vi "Compile with Data.vi"(6 "Loader":refnum<class "Loader.lvclass">, 7 "Data":refnum<class "Datum.lvclass">=refnum, 8 "Error In":errorcluster, 11 "Input":string) -> (0 "Error Out":errorcluster, 3 "Output":string)   [LabVIEW 2018, in "Toolkit.lvlib"]
doc: "Compile a Mustache template as a string using the types of data passed into the compiler to control the how and what is provided in the output. The type fo data for each tag and key can determine the rendering behavior of the node in the syntax tree, so LabVIEW classes are provided to represent the different types of data."
uses:
  Toolkit.lvlib
  Data/Datum/Datum.lvclass
  Data/Map/Map.lvclass
  Low-Level/Loaders/Loader/Loader.lvclass
  Low-Level/Support/Lex String.vi
  Low-Level/Support/Render to String.vi
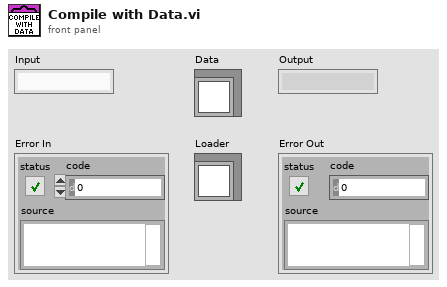
[diagram p1: front panel]
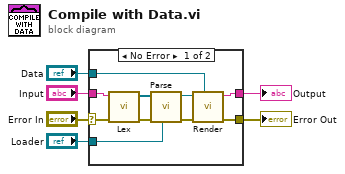
[diagram p0: block diagram]
diagram:
  n1 = case shown="No Error" "Error In" {
    selector: "Error In" -> [w10 w17]
    tunnel: [w13 w17] -> w6
    tunnel: "Input" -> [w9 w18]
    tunnel: [w12 w18] -> w4
    tunnel: "Data" -> [w11 _]
    tunnel: "Loader" -> [w7 _]
    frame No Error {
      n2 = call-poly "Lex.vi"("Error In"=w10, "Input"=w9) -> ("Error Out"=w8:errorcluster, "Tokens"=w16:refnum<class "Token.lvclass">[])  [unwired: 8 in]
      n3 = call "Parse.vi"("Loader"=w7, "Error In"=w8, "Tokens"=w16) -> ("Error Out"=w14:errorcluster, "Abstract Syntax Tree"=w15:refnum<class "Root.lvclass">)  [unwired: 7 in]
      n4 = call-poly "Render.vi"("Data"=w11, "Error In"=w14, "Abstract Syntax Tree"=w15) -> ("Error Out"=w13:errorcluster, "Output"=w12:string)  [unwired: 7 in]
    }
    frame Error {
    }
  }
  "Error Out" <- w6
  "Output" <- w4
